vi "direct_ref_dp_sat_dT_T.vi"(8 "Error (Input)":errorcluster, 10 "Temperature in K (Input)":dbl, 11 "WorkingPair (Input)":T1={"no_iso"=1, "no_p_sat"=1, "path_db"="D:\\Driesel\\SorpLibLocal\\LabVIEW_wrapper\\data\\json\\sorpproplib_minimalExample.json", "wp_as"="silicagel", "wp_st"="123", "wp_iso"="DubininArctan1", "wp_rf"="water", "rf_rhol"="SaturatedLiquidDensity_EoS1", "no_rhol"=1, "rf_psat"="VaporPressure_EoS1"}) -> (0 "Error (Output)":errorcluster, 3 "Der. of saturation pressure wrt temperature in Pa/K (Output)":dbl)   [LabVIEW 2017]
doc: "direct_ref_dp_sat_dT_T:\n * -----------------------\n *\n * Calculates derivative of saturation pressure in Pa/K wrt to temperature\n * depending on equilibrium temperature T in K.\n *\n * Parameters:\n * -----------\n * double T_K:\n * Equilibrium temperature in K.\n *\n * const char *path_db:\n * Path to database.\n * const char *wp_as:\n * Name of sorbent.\n * const char *wp_st:\n * Name of sub-type of sorbent.\n * const char *wp_rf:\n * Name of refrigerant.\n * const char *wp_iso:\n * Name of isotherm.\n * int no_iso:\n * ID of isotherm (i.e. when more than one isotherm is available)\n * const char *rf_psat:\n * Name of calculation approach for vapor pressure.\n * int no_p_sat:\n * ID of vapor pressure equation (i.e. when more than one equation is\n * available)\n * const char *rf_rhol:\n * Name of calculation approach for liquid density.\n * int no_rhol:\n * ID of liquid density equation (i.e. when more than one equation is\n * available)\n *\n * Returns:\n * --------\n * double:\n * Derivative of saturation pressure wrt temperature in Pa/K.\n *\n * History:\n * --------\n *12/07/2021, by Jannik Driesel (supervised by Mirko Engelpracht)\n * First implementation."
uses:
  data/win32bit/libsorpPropLib.dll
panel:
  # "Path to database"
  # "Name of sorbent"
  # "Name of sub-type of sorbent"
  # "Name of refrigerant"
  # "Name of isotherm"
  # "ID of isotherm"
  # "Name of calculation approach for vapor pressure"
  # "ID of vapor pressure equation"
  # "Name of calculation approach for liquid density"
  # "ID of liquid density equation"
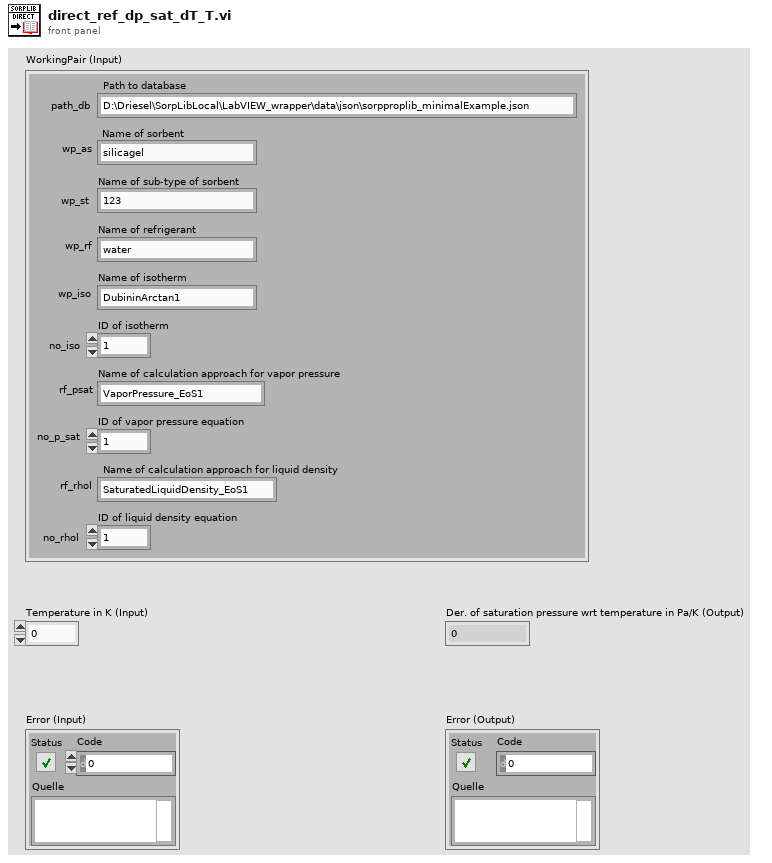
[diagram p1: front panel]
types:
  T1 = cluster{"no_iso":i32, "no_p_sat":i32, "path_db":string, "wp_as":string, "wp_st":string, "wp_iso":string, "wp_rf":string, "rf_rhol":string, "no_rhol":i32, "rf_psat":string}
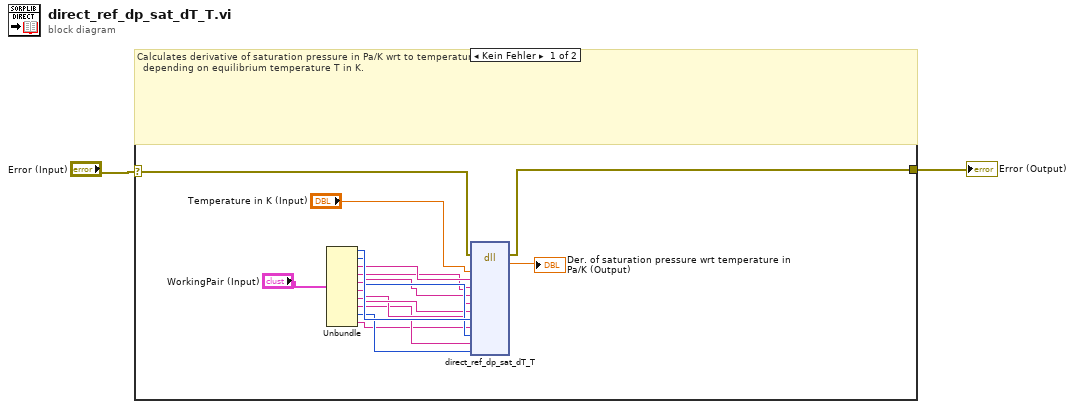
[diagram p0: block diagram]
diagram:
  n1 = case shown="Kein Fehler" "Error (Input)" {
    selector: "Error (Input)" -> [w16 w18]
    tunnel: [w15 w18] -> w2
    frame No Error {
      # "Calculates derivative of saturation pressure in Pa/K wrt to temperature\n  depending on equilibrium temperature T in K."
      n2 = Unbundle("WorkingPair (Input)") -> ("no_iso"=w13:i32, "no_p_sat"=w12:i32, "path_db"=w11:string, "wp_as"=w10:string, "wp_st"=w9:string, "wp_iso"=w8:string, "wp_rf"=w7:string, "rf_rhol"=w6:string, "no_rhol"=w5:i32, "rf_psat"=w4:string)
      n3 = dll-call lib="D:/Driesel/SorpLibLocal/LabVIEW_wrapper/data/win32bit/libsorpPropLib.dll" fn="direct_ref_dp_sat_dT_T"(error in=w16, "T_K"="Temperature in K (Input)", "path_db"=w11, "wp_as"=w10, "wp_st"=w9, "wp_rf"=w7, "wp_iso"=w8, "no_iso"=w13, "rf_psat"=w4, "no_p_sat"=w12, "rf_rhol"=w6, "no_rhol"=w5) -> (error out=w15:errorcluster, "dp_sat_dT"=→"Der. of saturation pressure wrt temperature in Pa/K (Output)":dbl)  [unwired: 13 in, 1 out]
    }
    frame Error {
      # "Error - No calculations"
    }
  }
  "Error (Output)" <- w2
